vi "Compile Connect Channel Data.vi"(8 "error in (no error)":errorcluster, 10 "Connect Chan Refs":T1[](array[typedef]) format="%.0x", 11 "Device ref":T1 format="%.0x") -> (0 "error out":errorcluster, 3 "Device ref dup":T1 format="%.0x", 5 "Compiled HW Channels":T2[](array[typedef]))   [LabVIEW 2023, in "NI 272x Resistive Simulation Custom Device Configuration.lvlib"]
uses:
  NI 272x Resistive Simulation Custom Device Configuration.lvlib
  <vilib>/NI VeriStand/Custom Device API/Custom Device Item Ref.ctl
  Controls/Compiled Connect Channel.ctl
  Globals/Names.vi
  <vilib>/NI VeriStand/Custom Device API/Get Item Property (I32).vi
  <vilib>/NI VeriStand/Custom Device API/Custom Device API.lvlib
  <vilib>/NI VeriStand/Custom Device Tools/Custom Device Utility Library/Custom Device Utility Library.lvlib
  NI 272x Resistive Simulation Custom Device Shared.lvlib
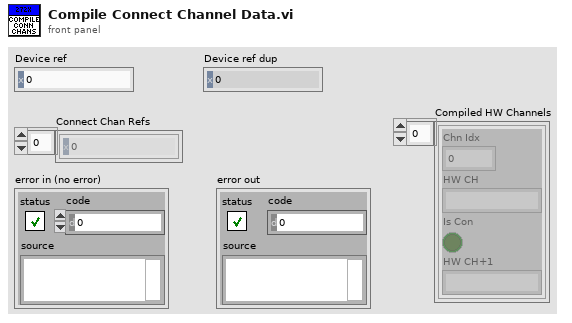
[diagram p1: front panel]
types:
  T1 = typedef "Custom Device API.lvlib/Custom Device Item Ref.ctl" = u64
  T2 = typedef "NI 272x Resistive Simulation Custom Device Shared.lvlib/Compiled Connect Channel.ctl" = cluster{"Chn Idx":i32, "HW CH":string, "Is Con":bool, "HW CH+1":string}
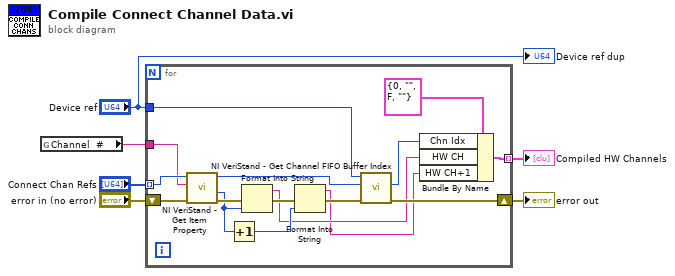
[diagram p0: block diagram]
diagram:
  n1 = global read "Names.vi" "Channel  #"() -> (w6:string)
  n2 = for {
    tunnel: "Connect Chan Refs" -> [w19] mode=indexing
    tunnel: w6 -> [w18]
    tunnel: "Device ref" -> [w14]
    shift-right: [w17] -> w3
    shift-left: "error in (no error)" -> [w22]
    tunnel: [w16] -> w2 mode=indexing
    n3 = call-poly <vilib>:"NI VeriStand - Get Item Property.vi"("error in (no error)"=w22, "Property Name"=w18, "Item Ref in"=w19) -> ("error out"=w20:errorcluster, "Value"=w10:i32, "Item Ref out"=w13:T1)  [unwired: 5 in, 1 out]
    n4 = Increment(x=w10) -> (x+1=w9:i32)
    n5 = Format Into String(error in=w20, w10) -> (resulting string=w8:string, error out=w12:errorcluster)  [unwired: 2 in]
    n6 = Format Into String(error in=w12, w9) -> (resulting string=w7:string, error out=w11:errorcluster)  [unwired: 2 in]
    n7 = call <vilib>:"NI VeriStand - Get Channel FIFO Buffer Index.vi"("error in"=w11, "Channel Ref"=w13, "Device Ref in"=w14) -> ("error out"=w17:errorcluster, "Channel FIFO Buffer Index"=w15:i32)  [unwired: 4 in, 3 out]
    n8 = Bundle By Name(cluster=T2 {"Chn Idx"=0, "HW CH"="", "Is Con"=FALSE, "HW CH+1"=""} ("Connect Chn"), "Chn Idx"=w15, "HW CH"=w8, "HW CH+1"=w7) -> (w16:T2)
  }
  "error out" <- w3
  "Compiled HW Channels" <- w2
  "Device ref dup" <- "Device ref"
